vi "Get Sheet Names.vi"(8 "error in":errorcluster, 11 "SpreadsheetDoc in":refnum<k24>) -> (0 "error out":errorcluster, 2 "Sheet Names":string[](array[string]), 3 "SpreadsheetDoc out":refnum<k24>)   [LabVIEW 2019, in "Open Xml.lvlib"]
uses:
  Open Xml.lvlib
  D:/git/Open-Xml-LabVIEW/Source/DocumentFormat.OpenXml.dll
  DocumentFormat.OpenXml.dll
  D:/git/Open-Xml-LabVIEW/Source/DocumentFormat.OpenXml.Framework.dll
  DocumentFormat.OpenXml.Framework.dll
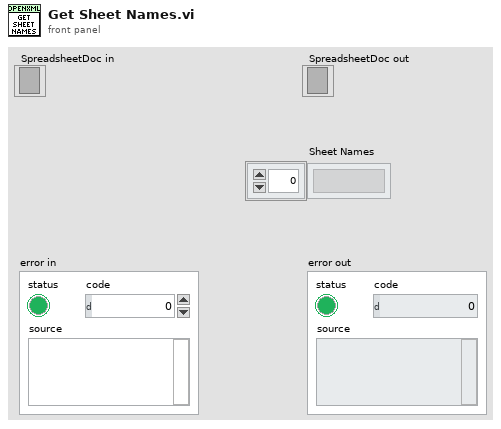
[diagram p1: front panel]
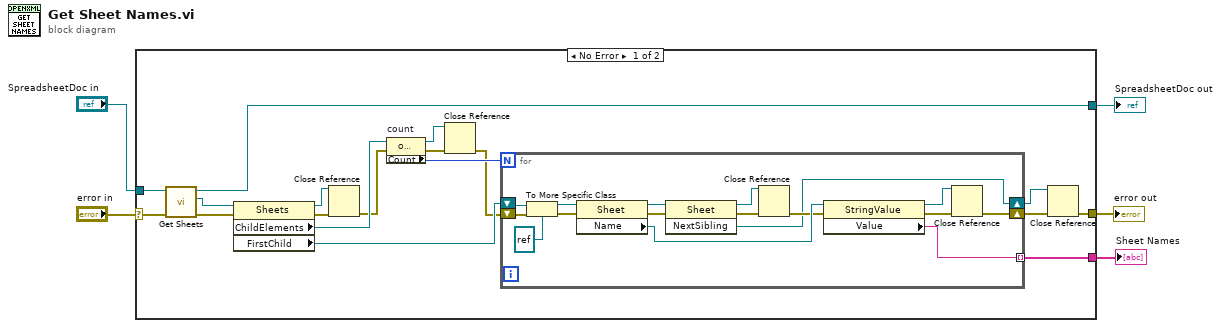
[diagram p0: block diagram]
diagram:
  n1 = case shown="No Error" "error in" {
    selector: "error in" -> [w23 w41]
    tunnel: "SpreadsheetDoc in" -> [w22 w40]
    tunnel: [w21 w40] -> w3
    tunnel: [w14 _] -> w2
    tunnel: [w7 w41] -> w1
    frame No Error {
      n2 = call "Get Sheets.vi"("error in"=w23, "SpreadsheetDocument in"=w22) -> ("error out"=w20:errorcluster, "Sheets"=w19:refnum<k24>, "SpreadsheetDocument out"=w21:refnum<k24>)  [unwired: 7 in]
      n3 = property class="Sheets"(reference=w19, error in=w20) -> (reference out=w12:refnum<k24>, error out=w11:errorcluster, "ChildElements"=w18:refnum<k24>, "FirstChild"=w16:refnum<k24>)
      n4 = Close Reference(reference=w12, error in (no error)=w11) -> (error out=w10:errorcluster)
      n5 = property on="count" class="OpenXmlElementList"(reference=w18, error in=w10) -> (reference out=w13:refnum<k24>, error out=w9:errorcluster, "Count"=w17:i32)
      n6 = Close Reference(reference=w13, error in (no error)=w9) -> (error out=w8:errorcluster)
      n7 = for {
        N: w17 -> [_]
        shift-right: [w30] -> w15
        shift-left: w8 -> [w39]
        tunnel: [w31] -> w14 mode=indexing
        shift-right: [w24] -> w6
        shift-left: w16 -> [w38]
        n8 = To More Specific Class(target class=refnum<k24> refnum ("FirstChild"), reference=w38, error in=w39) -> (specific class reference=w34:refnum<k24>, error out=w36:errorcluster)
        n9 = property class="Sheet"(reference=w34, error in=w36) -> (reference out=w26:refnum<k24>, error out=w35:errorcluster, "Name"=w32:refnum<k24>)
        n10 = invoke class="Sheet" method="NextSibling"(reference=w26, error in=w35) -> (reference out=w25:refnum<k24>, error out=w27:errorcluster, "NextSibling"=w24:refnum<k24>)  [unwired: 1 in]
        n11 = Close Reference(reference=w25, error in (no error)=w27) -> (error out=w28:errorcluster)
        n12 = property class="StringValue"(reference=w32, error in=w28) -> (reference out=w29:refnum<k24>, error out=w33:errorcluster, "Value"=w31:string)
        n13 = Close Reference(reference=w29, error in (no error)=w33) -> (error out=w30:errorcluster)
      }
      n14 = Close Reference(reference=w6, error in (no error)=w15) -> (error out=w7:errorcluster)
    }
    frame Error {
    }
  }
  "error out" <- w1
  "SpreadsheetDoc out" <- w3
  "Sheet Names" <- w2
